vi "new.vi"(8 "error in (no error)":errorcluster) -> (0 "error out":errorcluster, 3 "NotifierStopMechanism out":refnum<class "NotifierStopMechanism.lvclass">)   [LabVIEW 2023, in "TLC_Daemon.lvlib" / "NotifierStopMechanism.lvclass"]
uses:
  NotifierStopMechanism.lvclass
  NotifierStopMechanism.lvclass/NotifierStopMechanism.ctl
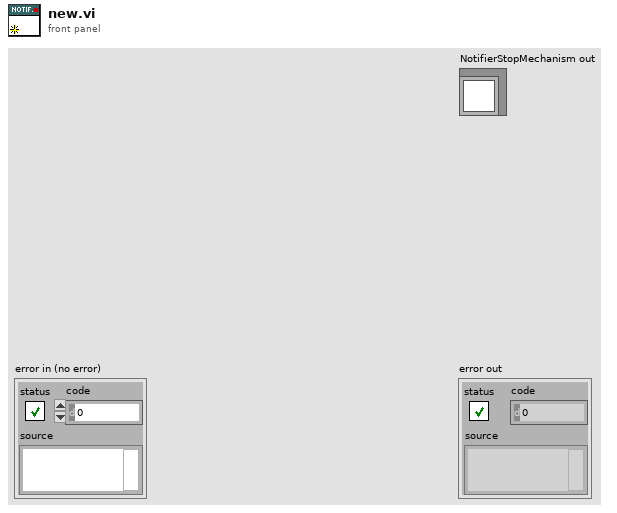
[diagram p1: front panel]
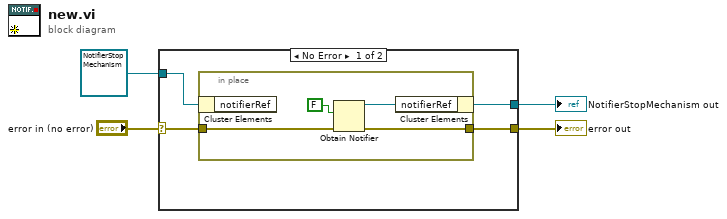
[diagram p0: block diagram]
diagram:
  n1 = case shown="No Error" "error in (no error)" {
    selector: "error in (no error)" -> [w8 w14]
    tunnel: [w7 w14] -> w3
    tunnel: [w5 w13] -> w1
    tunnel: refnum<class "NotifierStopMechanism.lvclass"> refnum ("NotifierStopMechanism in") -> [w6 w13]
    frame No Error {
      n2 = in-place {
        in-place-border: w8 -> [w11]
        in-place-border: [w10] -> w7
        n3 = in-place-cluster #1(w6) -> ()  [unwired: 1 out]
        n4 = Obtain Notifier(notification data type=FALSE, error in (no error)=w11) -> (notifier out=w9:refnum<notifier>, error out=w10:errorcluster)  [unwired: 2 in, 1 out]
        n5 = in-place-cluster #1("notifierRef"=w9) -> (w5:refnum<class "NotifierStopMechanism.lvclass">)
      }
    }
    frame Error {
    }
  }
  "error out" <- w3
  "NotifierStopMechanism out" <- w1
